vi "Get Motor Setpoint.vi"   [LabVIEW 2017, in "NI_Robotics_Motor Communication.lvclass"]
doc: "Returns the angles or angular velocity setpoints from the motor communication session. You must manually select the polymorphic instance to use."
uses:
  <vilib>/robotics/Actuation/Motor Communication/NI_Robotics_Motor Communication.lvclass
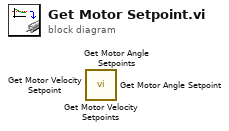
[diagram p0: block diagram]
diagram:
  n1 = call <vilib>:"Get Motor Velocity Setpoints.vi"() -> ()  [unwired: 8 in, 4 out]
  n2 = call <vilib>:"Get Motor Angle Setpoints.vi"() -> ()  [unwired: 8 in, 4 out]
  n3 = call <vilib>:"Get Motor Velocity Setpoint.vi"() -> ()  [unwired: 8 in, 4 out]
  n4 = call <vilib>:"Get Motor Angle Setpoint.vi"() -> ()  [unwired: 8 in, 4 out]
